vi "Format Client Request (Auto-Increment).vi"(8 "error in (no error)":errorcluster, 9 "initial string":string, 10 "JSON Value in":variant, 11 "method":string) -> (0 "error out":errorcluster, 2 "Request String":string)   [LabVIEW 2020, in "JSON-RPC Lib.lvlib" / "JSONRPC Client.lvclass"]
uses:
  JSONRPC Client.lvclass
  Variant Data Manipulation/Insert Element at Start.vi
  Variant Data Manipulation/Variant Data Manipulation.lvlib
  Variant JSON API/Variant JSON API.lvlib
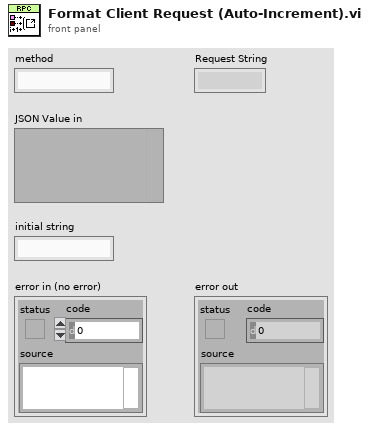
[diagram p1: front panel]
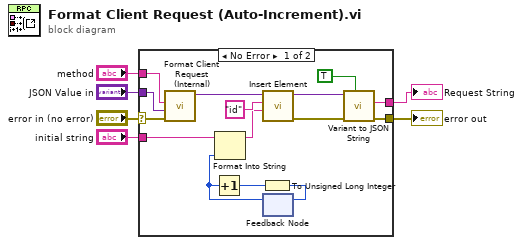
[diagram p0: block diagram]
diagram:
  n1 = case shown="No Error" "error in (no error)" {
    selector: "error in (no error)" -> [w21 w22]
    tunnel: [w10 w22] -> w5
    tunnel: "JSON Value in" -> [w19 _]
    tunnel: "method" -> [w20 _]
    tunnel: "initial string" -> [w18 _]
    tunnel: [w11 _] -> w1
    frame No Error {
      n2 = call "Format Client Request (Internal).vi"("error in (no error)"=w21, "params"=w19, "method"=w20) -> ("JSON Value out"=w12:variant)  [unwired: 7 in, 1 out]
      n3 = feedback #1() -> (w17:u32)  [unwired: 1 in]
      n4 = Increment(x=w17) -> (x+1=w16:u32)
      n5 = Format Into String(initial string=w18, w17) -> (resulting string=w7:string)  [unwired: 2 in, 1 out]
      n6 = To Unsigned Long Integer(number=w16) -> (unsigned 32bit integer=w15:u32)
      n7 = call-poly "Insert Element.vi"("element"=w7, "Name"="id", "Variant (Cluster) in"=w12) -> ("error out"=w13:errorcluster, "Variant (Cluster) out"=w14:variant)  [unwired: 7 in]
      n8 = feedback-in #1(w15) -> ()
      n9 = call "Variant to JSON String.vi"("pretty print? (F)"=TRUE ("pretty print? (T)"), "error in (no error)"=w13, "Variant in"=w14) -> ("error out"=w10:errorcluster, "String"=w11:string)  [unwired: 6 in, 1 out]
    }
    frame Error {
    }
  }
  "error out" <- w5
  "Request String" <- w1
